vi "Q -- range multiplier -- real.vi"(6 "factor":dbl=1.1, 10 "lower":dbl=-inf, 11 "upper":dbl=inf) -> (0 "center":dbl, 1 "window":dbl, 2 "lower OUT":dbl, 3 "upper OUT":dbl)   [LabVIEW 2015]
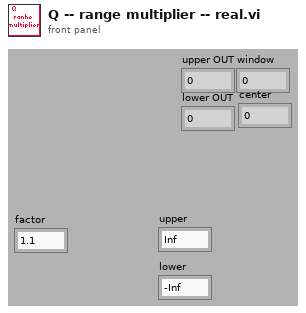
[diagram p1: front panel]
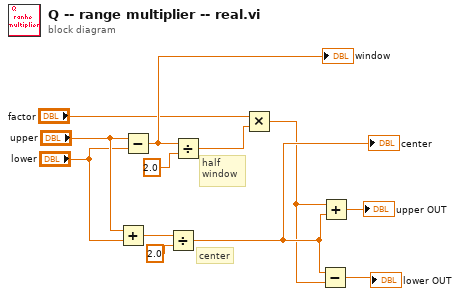
[diagram p0: block diagram]
diagram:
  # "half\nwindow"
  # "center"
  n1 = Add(x="upper", y="lower") -> (x+y=w8:dbl)
  n2 = Subtract(x="upper", y="lower") -> (x-y=w11:dbl)
  "window" <- w11
  n3 = Divide(x=w8, y=2.0) -> (x/y=w4:dbl)
  "center" <- w4
  n4 = Divide(x=w11, y=2.0) -> (x/y=w5:dbl)
  n5 = Multiply(x="factor", y=w5) -> (x*y=w3:dbl)
  n6 = Subtract(x=w4, y=w3) -> (x-y=→"lower OUT":dbl)
  n7 = Add(x=w3, y=w4) -> (x+y=→"upper OUT":dbl)
